vi "gameboard.size.vi"(7 "gameboard ref":refnum<vi>, 8 "error in (no error)":errorcluster, 11 "Worder in":refnum<class "Worder.lvclass">) -> (0 "error out":errorcluster, 3 "Worder out":refnum<class "Worder.lvclass">)   [LabVIEW 2020, in "Worder.lvclass"]
uses:
  Worder.lvclass
  Worder.lvclass/Worder.ctl
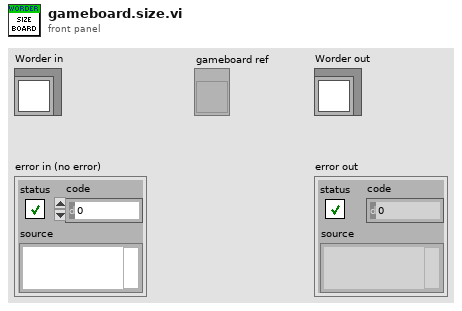
[diagram p1: front panel]
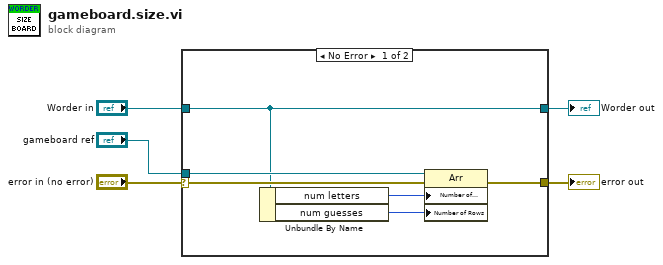
[diagram p0: block diagram]
diagram:
  n1 = case shown="No Error" "error in (no error)" {
    selector: "error in (no error)" -> [w10 w13]
    tunnel: [w9 w13] -> w4
    tunnel: [w8 w12] -> w2
    tunnel: "Worder in" -> [w8 w12]
    tunnel: "gameboard ref" -> [w11 _]
    frame No Error {
      n2 = Unbundle By Name(w8) -> ("num letters"=w7:i32, "num guesses"=w6:i32)
      n3 = property class="Arr"(reference=w11, error in=w10, "Number of Columns"=w7, "Number of Rows"=w6) -> (error out=w9:errorcluster)  [unwired: 1 out]
    }
    frame Error {
    }
  }
  "error out" <- w4
  "Worder out" <- w2
